vi "read_G2SEM.vi"(5 "folder_base":string="z:\\e1039_data\\slowcontrol_data", 6 "wait":i32=10, 7 "name":string="S:G2SEM", 8 "date_time":timestamp, 11 "spill_id":i32=1908144) -> (0 "found":bool, 3 "G2SEM":dbl format="%#_6e")   [LabVIEW 2019]
uses:
  <vilib>/Utility/file.llb/Read Delimited Spreadsheet (string).vi
panel:
  out "waiting":i32
  out "file_path":string
  # "VI to read the G2SEM value from TSV files recorded by the E1039 slow-control program.\nIt is supposed to find the value in real time, namely the spill specified by \"spill_id\" is of today.\nIf so, \"date_time\" can be unwired.  If not, it has to be wired to specify the date of the spill."
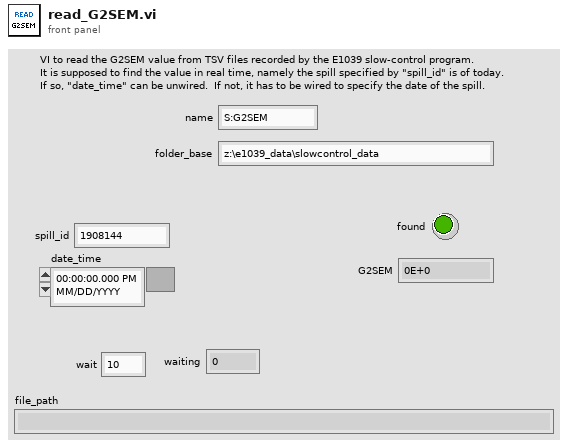
[diagram p1: front panel]
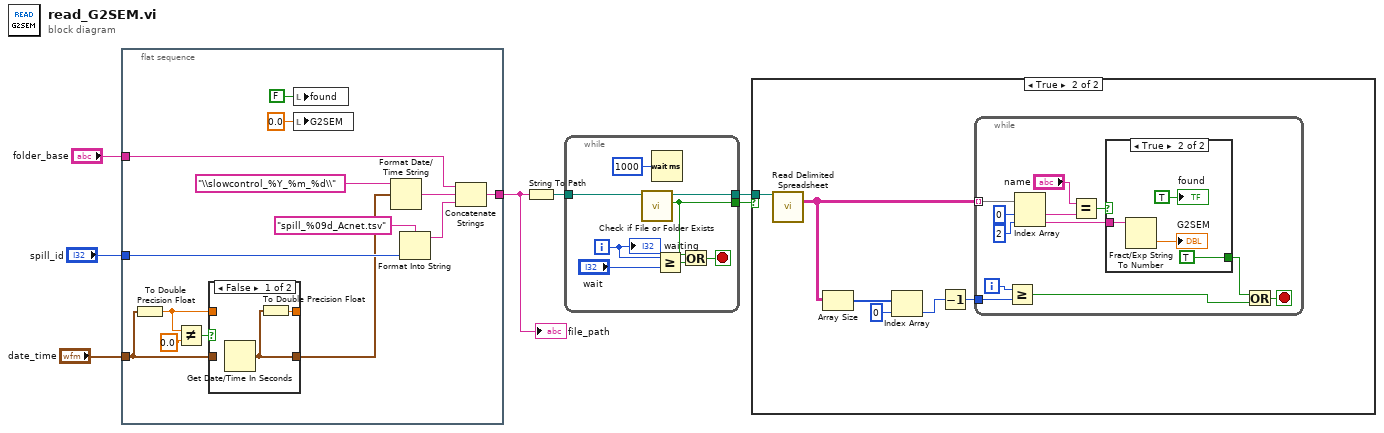
[diagram p0: block diagram]
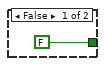
[diagram p4: hidden frame]
diagram:
  n1 = flat-sequence {
    tunnel: "date_time" -> [w18]
    tunnel: "spill_id" -> [w15]
    tunnel: "folder_base" -> [w14]
    tunnel: [w10] -> w1
    frame #0 {
      n2 = To Double Precision Float(number=w18) -> (double precision float=w19:dbl)
      n3 = Not Equal?(x=w19, y=0.0) -> (x != y?=w21:bool)
      n4 = case shown="False" w21 {
        tunnel: [w22 w25] -> w11
        tunnel: w18 -> [_ w25]
        tunnel: [w23 w24] -> _
        tunnel: w19 -> [_ w24]
        frame False {
          n5 = Get Date/Time In Seconds() -> (seconds since 1Jan1904=w22:timestamp)
          n6 = To Double Precision Float(number=w22) -> (double precision float=w23:dbl)
        }
        frame True {
        }
      }
      n7 = local write "found"(FALSE ("found")) -> ()
      n8 = local write "G2SEM"(0.0 ("G2SEM")) -> ()
      n9 = Format Date/Time String(time format string (%c)="\\slowcontrol_%Y_%m_%d\\", seconds (now)=w11) -> (date/time string=w13:string)  [unwired: 1 in]
      n10 = Format Into String(format string="spill_%09d_Acnet.tsv", w15) -> (resulting string=w12:string)  [unwired: 2 in, 1 out]
      n11 = Concatenate Strings(w14, w13, w12) -> (w10:string)
    }
  }
  n12 = String To Path(string=w1) -> (path=w4:path)
  n13 = while {
    tunnel: w4 -> [w33]
    tunnel: [w28] -> w2
    tunnel: [w27] -> w3
    i -> [w29]
    stop <- w32 stop-if-true
    n14 = call <vilib>:"Check if File or Folder Exists.vi"("path"=w33) -> ("file or folder exists?"=w28:bool, "dup path"=w27:path)  [unwired: 8 in, 1 out]
    n15 = Wait (ms)(milliseconds to wait=u32 1000) -> ()  [unwired: 1 out]
    n16 = Greater Or Equal?(x=w29, y="wait") -> (x >= y?=w31:bool)
    n17 = Or(x=w28, y=w31) -> (x .or. y?=w32:bool)
    "waiting" <- w29
  }
  n18 = case shown="True" w2 {
    tunnel: w3 -> [_ w39]
    frame False {
    }
    frame True {
      n19 = call-poly <vilib>:"Read Delimited Spreadsheet.vi"("file path (dialog if empty)"=w39) -> ("all rows"=w38:string[][])  [unwired: 9 in, 5 out]
      n20 = Array Size(array=w38) -> (size(s)=w36:i32[])
      n21 = Index Array(array=w36, index=0) -> (element=w34:i32)
      n22 = Decrement(x=w34) -> (x-1=w37:i32)
      n23 = while {
        tunnel: w38 -> [w51] mode=indexing
        tunnel: w37 -> [w44]
        i -> [w43]
        stop <- w42 stop-if-true
        n24 = Greater Or Equal?(x=w43, y=w44) -> (x >= y?=w41:bool)
        n25 = Index Array(array=w51, index #1=0 ("index"), index #2=2 ("index")) -> (element #1=w49:string, element #2=w45:string)
        n26 = Equal?(x="name", y=w49) -> (x = y?=w47:bool)
        n27 = case shown="True" w47 {
          tunnel: w45 -> [_ w56]
          tunnel: [FALSE TRUE] -> w40
          frame False {
          }
          frame True {
            n28 = Fract/Exp String To Number(string=w56) -> (number=→"G2SEM":dbl)  [unwired: 3 in, 1 out]
            "found" <- TRUE ("found")
          }
        }
        n29 = Or(x=w40, y=w41) -> (x .or. y?=w42:bool)
      }
    }
  }
  "file_path" <- w1
